vi "公式节点习题.vi"() -> ()   [LabVIEW 2017]
panel:
  out "波形图":dbl[][](graph)
  in  "a":dbl
  in  "b":dbl
  out "y2":dbl
  out "y1":dbl
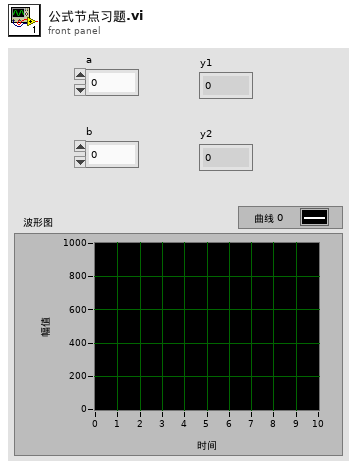
[diagram p1: front panel]
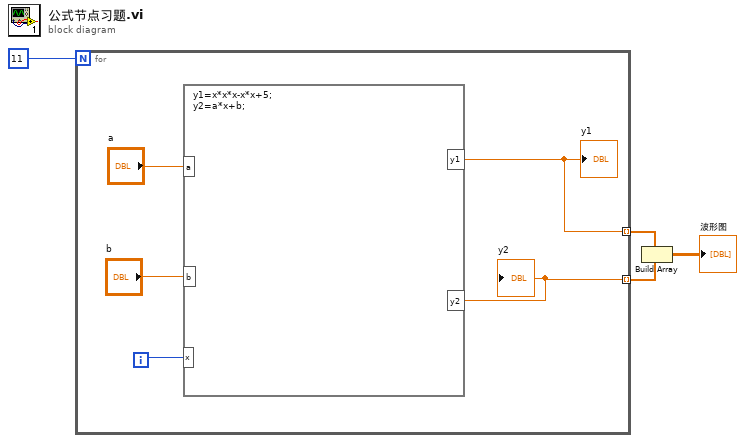
[diagram p0: block diagram]
diagram:
  n1 = for {
    N: 11 ("数值") -> [_]
    tunnel: [w9] -> w4 mode=indexing
    tunnel: [w8] -> w3 mode=indexing
    i -> [w5]
    n2 = formula code="y1=x*x*x-x*x+5;\ny2=a*x+b;"("a"="a", "b"="b", "x"=w5) -> ("y1"=w9:dbl, "y2"=w8:dbl)
    "y1" <- w9
    "y2" <- w8
  }
  n3 = Build Array(w4, w3) -> (→"波形图":dbl[][])
